vi "Gripper Controller.vi"(8 "error in":errorcluster) -> ()   [LabVIEW 2017]
doc: "This VI executes continuously carrying out the current operation and responding to updates or new operations. It will often contain the timing or control code that is difficult to place directly in TeleOp. This VI generally opens all sensors and motors and isolates the rest of the robot code from knowing how the operations are carried out."
uses:
  Gripper Operations.ctl
  Gripper Setpoints.ctl
  <vilib>/Rock Robotics/WPI/SafetyOutput/WPI_SafetyOutputConfigMenu.ctl
  <vilib>/Rock Robotics/SystemInterfaces/DIO/FPGA_DIOPWMChannel.ctl
  <vilib>/Rock Robotics/WPI/MotorControl/WPI_MotorControlOpen TalonSRX.vi
  <vilib>/Rock Robotics/WPI/RobotDrive/WPI_RobotDriveOpen2MotorWithExistingMotors.vi
  <vilib>/Rock Robotics/WPI/MotorControl/WPI_MotorControlOpen Talon.vi
  <vilib>/Rock Robotics/Network Tables/NT Write Boolean.vi
  <vilib>/Rock Robotics/WPI/Framework/Completion Status.ctl
panel:
  in  "Interactive Values":T1
  out "Current\nCmd":string
  in  "Buttons":cluster{"Execute Cmd":bool, "Abort Cmd":bool}
  out "Command Timing":cluster{"Start Time (ms)":u32, "Iterations":i32}
  out "Status":T3
  # "Tip: It may be helpful to observe inputs and sensor values.\nYou may also want to display tuning or debugging controls."
  # "Interactive Command: You may fill in the settings for a command\nand schedule it with the Execute button. You can observe and abort\nany command while fine tuning the code for the controller."
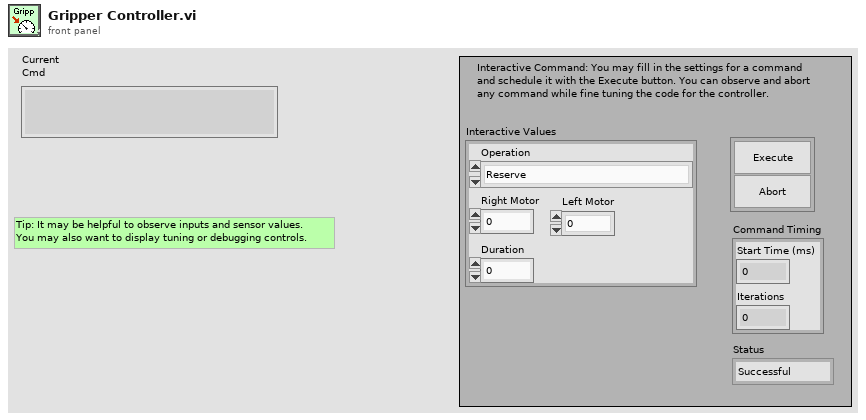
[diagram p1: front panel]
types:
  T1 = typedef "Gripper Setpoints.ctl" = cluster{"Operation":T2, "Right Motor":dbl, "Duration":dbl, "Left Motor":dbl}
  T2 = typedef "Gripper Operations.ctl" = enum16{"Reserve", "Read Current", "Immediate", "Set Gripper Motors", "Gripper Drive For Time"}
  T3 = typedef "Completion Status.ctl" = enum16{"Successful", "Aborted", "Incomplete"}
  T4 = typedef "FPGA_DIOPWMChannel.ctl" = enum8{"PWM 0", "PWM 1", "PWM 2", "PWM 3", "PWM 4", "PWM 5", "PWM 6", "PWM 7", "PWM 8", "PWM 9", "PWM MXP 0", "PWM MXP 1", "PWM MXP 2", "PWM MXP 3", "PWM MXP 4", "PWM MXP 5", "PWM MXP 6", "PWM MXP 7", "PWM MXP 8", "PWM MXP 9", "Invalid"}
  T5 = typedef "WPI_SafetyOutputConfigMenu.ctl" = enum16{"Enable", "Disable"}
  T6 = typedef "WPI_MotorControlDeviceRef.ctl" = cluster{"DeviceStatus":errorcluster, "Type":T7, "PWM":cluster{"PWM Channel":T4, "DeadBand":T8}, "CAN":cluster{"Device Number":u8, "SetOutput VI Ref":variant, "GetOutput VI Ref":variant, "Enable VI Ref":variant, "Disable VI Ref":variant, "Data":variant}, "Invert":bool, "DIO PWM":cluster{"PWM \"Enable\" Channel":T4, "DIOChannel":T9, "PWM Rate":dbl}}
  T7 = typedef "WPI_MotorControlType.ctl" = enum16{"PWM", "CAN", "DIO PWM"}
  T8 = typedef "WPI_PWMDeadband.ctl" = cluster{"Name":string, "maxPositivePwm":i32, "minPositivePwm":i32, "centerPwm":i32, "maxNegativePwm":i32, "minNegativePwm":i32, "angularRange":u16}
  T9 = typedef "FPGA_DIOChannel.ctl" = enum8{"DIO 0", "DIO 1", "DIO 2", "DIO 3", "DIO 4", "DIO 5", "DIO 6", "DIO 7", "DIO 8", "DIO 9", "DIO MXP 0", "DIO MXP 1", "DIO MXP 2", "DIO MXP 3", "DIO MXP 4", "DIO MXP 5", "DIO MXP 6", "DIO MXP 7", "DIO MXP 8", "DIO MXP 9", "DIO MXP 10", "DIO MXP 11", "DIO MXP 12", "DIO MXP 13", "DIO MXP 14", "DIO MXP 15", "SPI Port CS1", "SPI Port CS2", "SPI Port CS3", "SPI Port MISO", "SPI Port MOSI", "Invalid"}
  T10 = typedef "WPI_RobotDriveDevRef.ctl" = cluster{"DevStatus":errorcluster, "Motors[]":T6[], "Square Inputs":bool, "Max Output":dbl}
  T11 = typedef "Command Status Info.ctl" = cluster{"Name":string, "Status":T3, "notifier out":T12}
  T12 = typedef "Completion Notifier.ctl" = refnum<notifier>
  T13 = cluster{"Current Command":T1, "Command Timing":cluster{"Start Time (ms)":u32, "Iterations":i32}, "Command Arguments":cluster{"Command Info":T11, "Description":string, "Default Command":T1, "queue out":refnum<queue>, "Subsystem Name":string}}
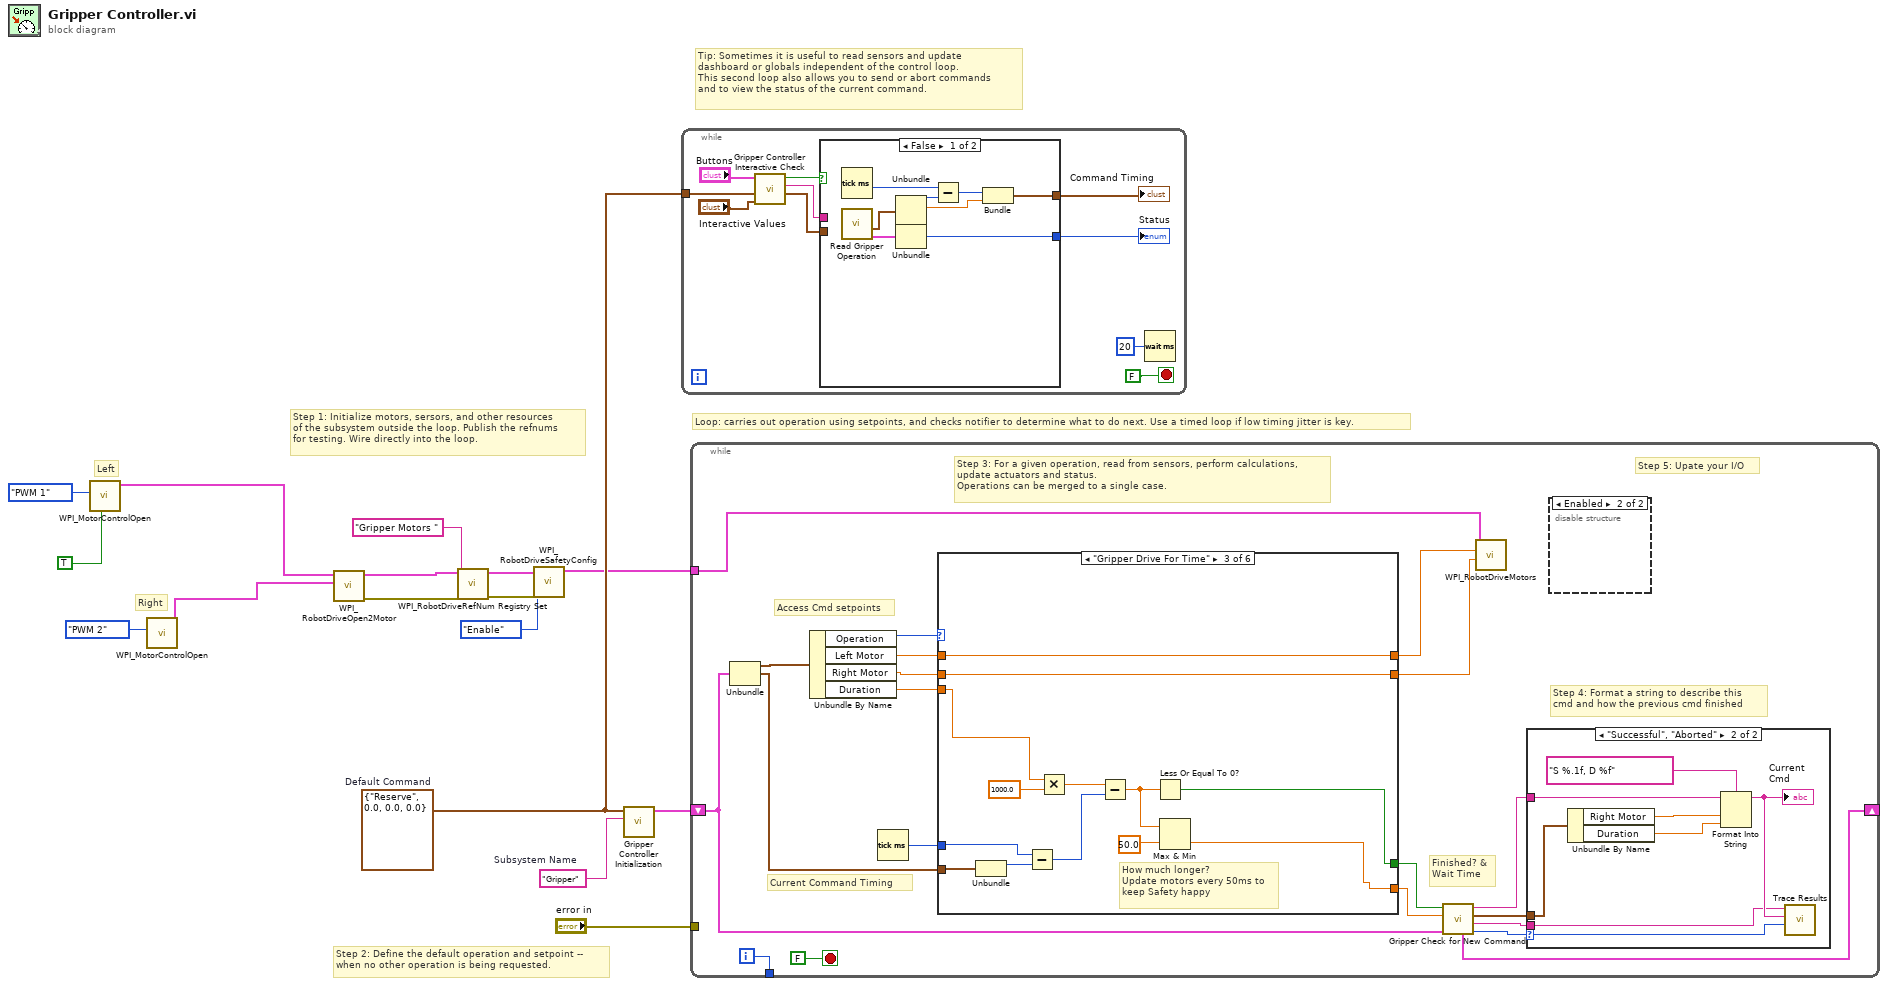
[diagram p0: block diagram]
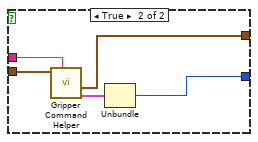
[diagram p2: hidden frame]
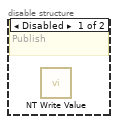
[diagram p3: hidden frame]
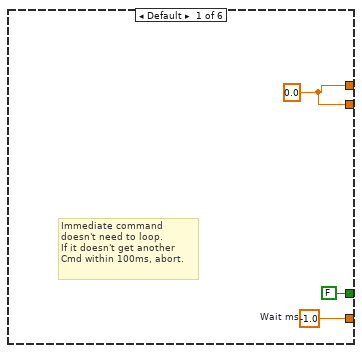
[diagram p5: hidden frame]
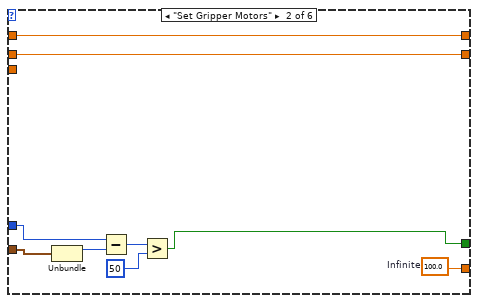
[diagram p6: hidden frame]
diagram:
  w13 = T1 {"Operation"=enum."Reserve", "Right Motor"=0.0, "Duration"=0.0, "Left Motor"=0.0}  # Default Command
  w14 = "Gripper"  # Subsystem Name
  # "Right"
  # "Left"
  # "Tip: Sometimes it is useful to read sensors and update\ndashboard or globals independent of the control loop.\nThis second loop also allows you to send or abort commands\nand to view the status of the current command."
  # "Step 2: Define the default operation and setpoint --\nwhen no other operation is being requested."
  # "Step 1: Initialize motors, sersors, and other resources\nof the subsystem outside the loop. Publish the refnums\nfor testing. Wire directly into the loop."
  # "Loop: carries out operation using setpoints, and checks notifier to determine what to do next. Use a timed loop if low timing jitter is key."
  n1 = call-poly <vilib>:"WPI_MotorControlOpen.vi"("Invert"=TRUE, "PWM Channel"=FPGA_DIOPWMChannel."PWM 1") -> ("MotorControlDeviceRef"=w12:T6)  [unwired: 8 in, 1 out]
  n2 = call-poly <vilib>:"WPI_MotorControlOpen.vi"("PWM Channel"=FPGA_DIOPWMChannel."PWM 2") -> ("MotorControlDeviceRef"=w11:T6)  [unwired: 9 in, 1 out]
  n3 = call-poly <vilib>:"WPI_RobotDriveOpen2Motor.vi"("Right Motor Dev Ref"=w11, "Left Motor Dev Ref"=w12) -> ("error out"=w7:errorcluster, "RobotDriveDevRef"=w10:T10)  [unwired: 8 in]
  n4 = call <vilib>:"WPI_RobotDriveRefNum Registry Set.vi"("error in (no error)"=w7, "refnum name"="Gripper Motors ", "RobotDriveDevRef"=w10) -> ("error out"=w5:errorcluster, "RobotDriveDevRef"=w6:T10)  [unwired: 7 in]
  n5 = call <vilib>:"WPI_RobotDriveSafetyConfig.vi"("error in (no error)"=w5, "mode"=WPI_SafetyOutputConfigMenu."Enable", "RobotDriveDevRef"=w6) -> ("RobotDriveDevRef"=w3:T10)  [unwired: 7 in, 1 out]
  n6 = call "Gripper Controller Initialization.vi"("Subsystem Name"=w14, "Default Command"=w13) -> ("Current Command"=w15:T13)  [unwired: 9 in]
  n7 = while {
    tunnel: w13 -> [w23]
    stop <- FALSE stop-if-true
    n8 = call "Gripper Controller Interactive Check.vi"("Interactive Command in"="Interactive Values", "Default Command"=w23, "Buttons"="Buttons") -> ("Interactive Command out"=w20:T1, "Trace String"=w21:string, "Schedule"=w22:bool)  [unwired: 6 in]
    n9 = case shown="False" w22 {
      tunnel: [w34 w39] -> w19
      tunnel: w20 -> [_ w37]
      tunnel: [w30 w35] -> w18
      tunnel: w21 -> [_ w38]
      frame False {
        n10 = Tick Count (ms)() -> (millisecond timer value=w29:u32)
        n11 = call "Read Gripper Operation.vi"() -> ("Command Info"=w27:T11, "SubSystem Data"=w28:T1)  [unwired: 9 in, 1 out]
        n12 = Unbundle(w28) -> ("Operation"=w33:T2, "Right Motor"=w31:dbl)  [unwired: 2 out]
        n13 = Unbundle(w27) -> ("Status"=w34:T3)  [unwired: 2 out]
        n14 = Subtract(x=w29, y=w33) -> (x-y=w32:u32)
        n15 = Bundle(w32, "Right Motor"=w31) -> (w30:cluster{u32, "Right Motor":dbl})  [unwired: 1 in]
      }
      frame True {
        n16 = call "Gripper Command Helper.vi"("Description"=w38, "SubSystem Data"=w37) -> ("Command Info Out"=w36:T11, "Command Timing"=w35:cluster{"Start Time (ms)":u32, "Iterations":i32})  [unwired: 7 in, 1 out]
        n17 = Unbundle(w36) -> ("Status"=w39:T3)  [unwired: 2 out]
      }
    }
    "Status" <- w19
    "Command Timing" <- w18
    n18 = Wait (ms)(milliseconds to wait=u32 20) -> ()  [unwired: 1 out]
  }
  n19 = while {
    shift-right: [w51] -> _
    shift-left: w15 -> [w44]
    tunnel: [w58] -> _
    tunnel: "error in" -> [_]
    tunnel: w3 -> [w43]
    i -> [w58]
    stop <- FALSE stop-if-true
    # "Step 5: Upate your I/O"
    # "Step 4: Format a string to describe this\ncmd and how the previous cmd finished"
    # "Current Command Timing"
    # "Access Cmd setpoints"
    # "Finished? &\nWait Time"
    # "Step 3: For a given operation, read from sensors, perform calculations,\nupdate actuators and status.\nOperations can be merged to a single case."
    n20 = Unbundle(w44) -> ("Current Command"=w57:T1, "Command Timing"=w53:cluster{"Start Time (ms)":u32, "Iterations":i32})  [unwired: 1 out]
    n21 = Unbundle By Name(w57) -> ("Operation"=w56:T2, "Left Motor"=w55:dbl, "Right Motor"=w52:dbl, "Duration"=w40:dbl)
    n22 = Tick Count (ms)() -> (millisecond timer value=w54:u32)
    n23 = case shown="\"Gripper Drive For Time\"" w56 {
      tunnel: [w70 w79 w80 _ _ _] -> w49
      tunnel: [FALSE w73 w81 _ _ _] -> w50
      tunnel: w53 -> [_ w76 w82 _ _ _]
      tunnel: w55 -> [_ w72 w92 _ _ _]
      tunnel: w54 -> [_ w75 w83 _ _ _]
      tunnel: w52 -> [_ w71 w91 _ _ _]
      tunnel: [w69 w72 w92 _ _ _] -> w42
      tunnel: [w69 w71 w91 _ _ _] -> w41
      tunnel: w40 -> [_ _ w84 _ _ _]
      frame Default {
        w69 = 0.0 ("Left Motor")
        w70 = -1.0  # Wait ms
        # "Immediate command\ndoesn't need to loop.\nIf it doesn't get another\nCmd within 100ms, abort."
      }
      frame "Set Gripper Motors" {
        w79 = 100.0  # Infinite
        n24 = Unbundle(w76) -> ("Start Time (ms)"=w74:u32)  [unwired: 1 out]
        n25 = Subtract(x=w75, y=w74) -> (x-y=w78:u32)
        n26 = Greater?(x=w78, y=u8 50 ("Left Motor")) -> (0:w73:bool)
      }
      frame "Gripper Drive For Time" {
        # "How much longer?\nUpdate motors every 50ms to\nkeep Safety happy"
        n27 = Unbundle(w82) -> ("Start Time (ms)"=w87:u32)  [unwired: 1 out]
        n28 = Subtract(x=w83, y=w87) -> (x-y=w90:u32)
        n29 = Multiply(x=w84, y=1000.0) -> (x*y=w89:dbl)
        n30 = Subtract(x=w89, y=w90) -> (x-y=w86:dbl)
        n31 = Less Or Equal To 0?(x=w86) -> (x <= 0?=w81:bool)
        n32 = Max & Min(x=w86, y=50.0) -> (min(x,y)=w80:dbl)  [unwired: 1 out]
      }
      frame "Immediate" {
      }
      frame "Read Current" {
      }
      frame "Reserve" {
      }
    }
    n33 = call "Gripper Check for New Command.vi"("Current Command"=w44, "Wait time (ms)"=w49, "Finished?"=w50) -> ("Completion"=w45:T3, "Subsystem Name"=w46:string, "Current Command"=w47:T1, "Initial Trace String"=w48:string, "NextCommand"=w51:T13)  [unwired: 4 in]
    n34 = call <vilib>:"WPI_RobotDriveMotors.vi"("RightSpeed"=w41, "LeftSpeed"=w42, "RobotDriveDevRef"=w43) -> ()  [unwired: 6 in, 3 out]
    n35 = case shown="\"Successful\", \"Aborted\"" w45 {
      selector: w45 -> [_ w67]
      tunnel: w48 -> [_ w63]
      tunnel: w47 -> [_ w64]
      tunnel: w46 -> [_ w60]
      frame "Incomplete", Default {
        # "Continuing current command"
      }
      frame "Successful", "Aborted" {
        # "Report and setup for next command"
        n36 = Unbundle By Name(w64) -> ("Right Motor"=w66:dbl, "Duration"=w61:dbl)
        n37 = Format Into String(format string="S %.1f, D %f", initial string=w63, w66, w61) -> (resulting string=w62:string)  [unwired: 1 in, 1 out]
        "Current\nCmd" <- w62
        n38 = call <vilib>:"Trace Results.vi"("Status of previous command"=w67, "Description"=w62, "Subsystem"=w60) -> ()  [unwired: 9 in]
      }
    }
    n39 = disable-structure shown="Enabled" {
      frame Disabled {
        # "Publish"
        n40 = call-poly <vilib>:"NT Write Value.vi"() -> ()  [unwired: 11 in, 1 out]
      }
      frame Enabled {
      }
    }
  }
